vi "Status Machine.vi"() -> ()   [LabVIEW 2018]
panel:
  in  "정지":bool
  in  "작업 3":bool
  in  "작업 2":bool
  in  "작업 1":bool
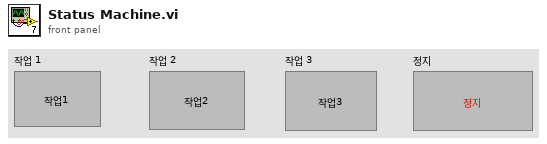
[diagram p1: front panel]
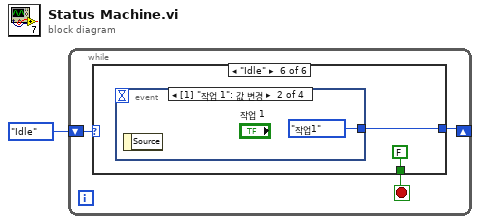
[diagram p0: block diagram]
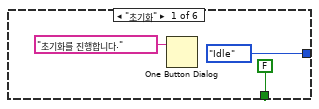
[diagram p2: hidden frame]
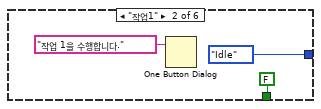
[diagram p3: hidden frame]
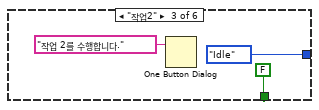
[diagram p4: hidden frame]
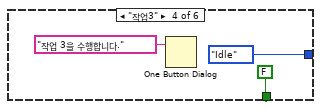
[diagram p5: hidden frame]
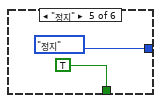
[diagram p6: hidden frame]
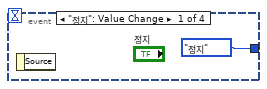
[diagram p7: hidden frame]
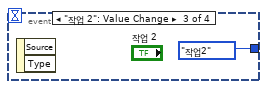
[diagram p8: hidden frame]
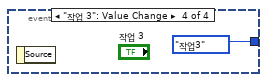
[diagram p9: hidden frame]
diagram:
  n1 = while {
    shift-right: [w3] -> _
    shift-left: enum16{"Idle", "초기화", "정지", "작업1", "작업2", "작업3"}."Idle" ("열거형") -> [w4]
    stop <- w2 stop-if-true
    n2 = case shown="\"Idle\"" w4 {
      tunnel: [enum16{"Idle", "초기화", "정지", "작업1", "작업2", "작업3"}."Idle" ("열거형") enum16{"Idle", "초기화", "정지", "작업1", "작업2", "작업3"}."Idle" ("열거형") enum16{"Idle", "초기화", "정지", "작업1", "작업2", "작업3"}."Idle" ("열거형") enum16{"Idle", "초기화", "정지", "작업1", "작업2", "작업3"}."Idle" ("열거형") enum16{"Idle", "초기화", "정지", "작업1", "작업2", "작업3"}."정지" ("열거형") w20] -> w3
      tunnel: [FALSE FALSE FALSE FALSE TRUE FALSE] -> w2
      frame "초기화" {
        n3 = One Button Dialog(message="초기화를 진행합니다." ("메시지")) -> ()  [unwired: 1 in, 1 out]
      }
      frame "작업1" {
        n4 = One Button Dialog(message="작업 1을 수행합니다." ("메시지")) -> ()  [unwired: 1 in, 1 out]
      }
      frame "작업2" {
        n5 = One Button Dialog(message="작업 2를 수행합니다." ("메시지")) -> ()  [unwired: 1 in, 1 out]
      }
      frame "작업3" {
        n6 = One Button Dialog(message="작업 3을 수행합니다." ("메시지")) -> ()  [unwired: 1 in, 1 out]
      }
      frame "정지" {
      }
      frame "Idle" {
        n7 = event shown="[1] \"작업 1\": 값 변경" {
          selector: _ -> [_ _ _ _]
          dyn-events: _ -> [_ _ _ _]
          timeout: _ -> [_ _ _ _]
          tunnel: [enum16{"Idle", "초기화", "정지", "작업1", "작업2", "작업3"}."정지" ("열거형") enum16{"Idle", "초기화", "정지", "작업1", "작업2", "작업3"}."작업1" ("열거형") enum16{"Idle", "초기화", "정지", "작업1", "작업2", "작업3"}."작업2" ("열거형") enum16{"Idle", "초기화", "정지", "작업1", "작업2", "작업3"}."작업3" ("열거형")] -> w20
          event "정지": Value Change {
            n8 = event-data() -> ()  [unwired: 1 in, 1 out]
          }
          event "작업 1": Value Change {
            n9 = event-data() -> ()  [unwired: 1 in, 1 out]
          }
          event "작업 2": Value Change {
            n10 = event-data() -> ()  [unwired: 1 in, 2 out]
          }
          event "작업 3": Value Change {
            n11 = event-data() -> ()  [unwired: 1 in, 1 out]
          }
        }
      }
    }
  }
